vi "Error Query.vi"(8 "error in (no error)":errorcluster, 11 "BH Druck PACE Series in":refnum<class "BH Druck PACE Series.lvclass">) -> (0 "error out":errorcluster, 3 "BH Druck PACE Series out":refnum<class "BH Druck PACE Series.lvclass">)   [LabVIEW 2022 SP3, in "BH Druck PACE Series.lvclass"]
uses:
  BH Druck PACE Series.lvclass
  BH Druck PACE Series.lvclass/BH Druck PACE Series.ctl
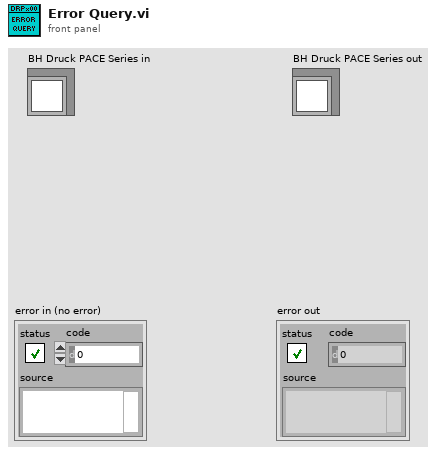
[diagram p1: front panel]
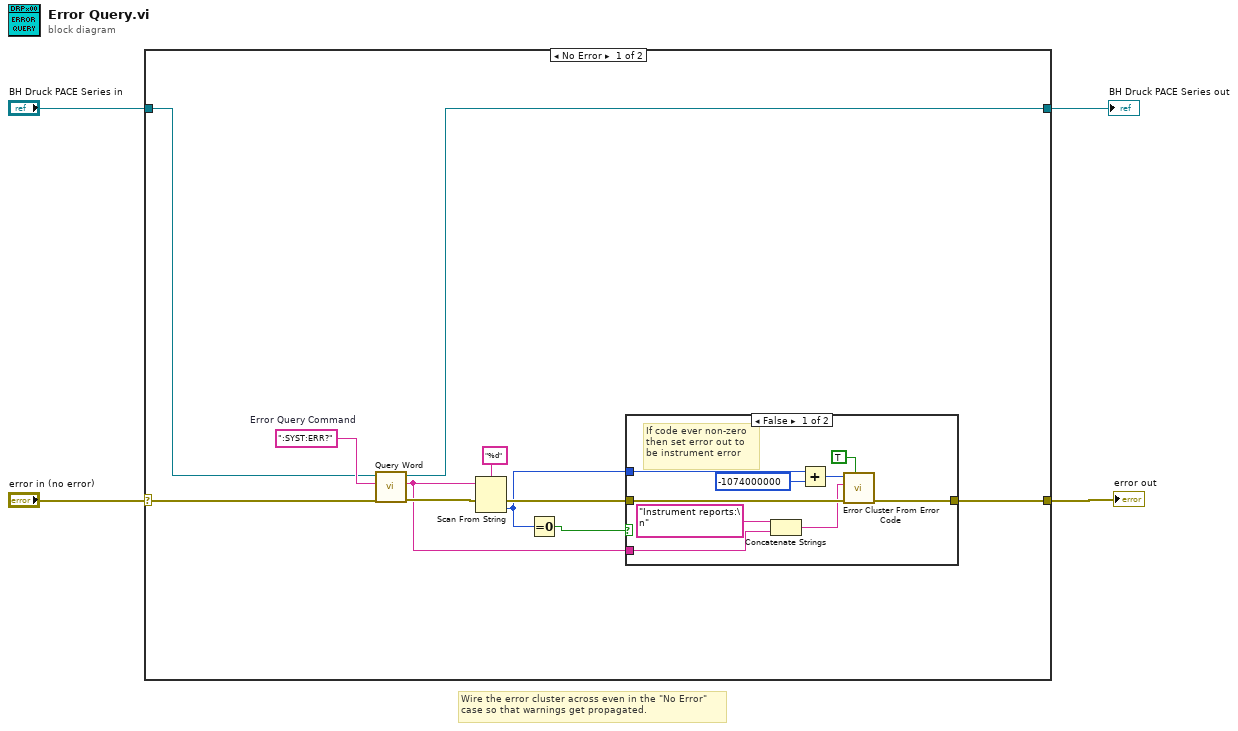
[diagram p0: block diagram]
diagram:
  # "Wire the error cluster across even in the \"No Error\"\ncase so that warnings get propagated."
  n1 = case shown="No Error" "error in (no error)" {
    selector: "error in (no error)" -> [w7 w27]
    tunnel: [w6 w27] -> w3
    tunnel: [w5 w26] -> w1
    tunnel: "BH Druck PACE Series in" -> [w8 w26]
    frame No Error {
      w12 = ":SYST:ERR?"  # Error Query Command
      n2 = call-dynamic "Query Word.vi"("error in (no error)"=w7, "Query String"=w12, "BH Druck PACE Series in"=w8) -> ("error out"=w10:errorcluster, "String Result"=w9:string, "BH Druck PACE Series out"=w5:refnum<class "BH Druck PACE Series.lvclass">)  [unwired: 6 in]
      n3 = Scan From String(format string="%d", input string=w9, error in=w10) -> (error out=w14:errorcluster, output 1=w11:i32)  [unwired: 2 in, 2 out]
      n4 = Equal To 0?(x=w11) -> (x = 0?=w13:bool)
      n5 = case shown="False" w13 {
        tunnel: [w23 w25] -> w6
        tunnel: w14 -> [w22 w25]
        tunnel: w9 -> [w17 _]
        tunnel: w11 -> [w20 _]
        frame False {
          # "If code ever non-zero\nthen set error out to\nbe instrument error"
          n6 = Concatenate Strings("Instrument reports:\n" ("Source"), w17) -> (w16:string)
          n7 = Add(x=w20, y=-1074000000 ("Code")) -> (x+y=w19:i32)
          n8 = call <vilib>:"Error Cluster From Error Code.vi"("show call chain? (False)"=TRUE, "error in (no error)"=w22, "error message (\"\")"=w16, "error code (0)"=w19) -> ("error out"=w23:errorcluster)  [unwired: 5 in]
        }
        frame True {
        }
      }
    }
    frame Error {
    }
  }
  "error out" <- w3
  "BH Druck PACE Series out" <- w1
